vi "ZyklussteuerungGV-01-17.vi"(0 "Traps/MachKoeff0":dbl[](array[numeric]), 1 "DIOsNummern":cluster{"DIOsMod2BNr":i32[]}[](array[cluster]), 2 "error in":errorcluster, 5 "Traps/MachKoeff1":dbl[](array[numeric]), 7 "ServosWarmHigh (us)KaltHigh(us)":T1, 9 "Traps/MachKoeff2":dbl[](array[numeric]), 11 "Schieberegister":T2, 12 "Zeitpunkte/Setpoints":T4 {"FPGAPID"."proportional gain (Kc)" format="%.11g"; "FPGAPID"."integral gain (Kc*Ts/Ti)" format="%.11g"; "FPGAPID"."derivative gain (Kc*Td/Ts)" format="%.11g"}, 13 "FPGA VI Reference In":refnum<k20>, 14 "MachKoeffs":T3) -> (4 "Schieberegister":T2, 8 "error out":errorcluster)   [LabVIEW 2010]
uses:
  <vilib>/rvi/interface/nirviReadWriteControl/nirviReadWriteControl.xnode
  C:/Users/HAGAR-IV/Desktop/Zeugs/markus/version feb 2012/FPGA Bitfiles/pertrasgcfpga2_FPGATarget_FPGA-Programm-01_A75D3647.lvbitx
  C:/Users/HAGAR-IV/Desktop/Zeugs/Johnny/pertrasgc fpga/FPGA-Programm-01-17.vi
  <vilib>/rvi/interface/common/niFpgaNodeNameForErrorReporting.ctl
  <vilib>/rvi/errors/niLvFpgaWhatHappensToTopLevelVI.ctl
  GVZwangs.vi
  GVHeizenLH.vi
  GVZeitenZyklen.vi
  GVZwangsMPV.vi
  GVZwangsMPVPos.vi
  GVVentilposition.vi
  GVHorstSP.vi
  <vilib>/Utility/error.llb/Error Cluster From Error Code.vi
  <vilib>/rvi/errors/niLvFpgaAdjustHostInterfaceError.vi
  NiFpgaLv.dll
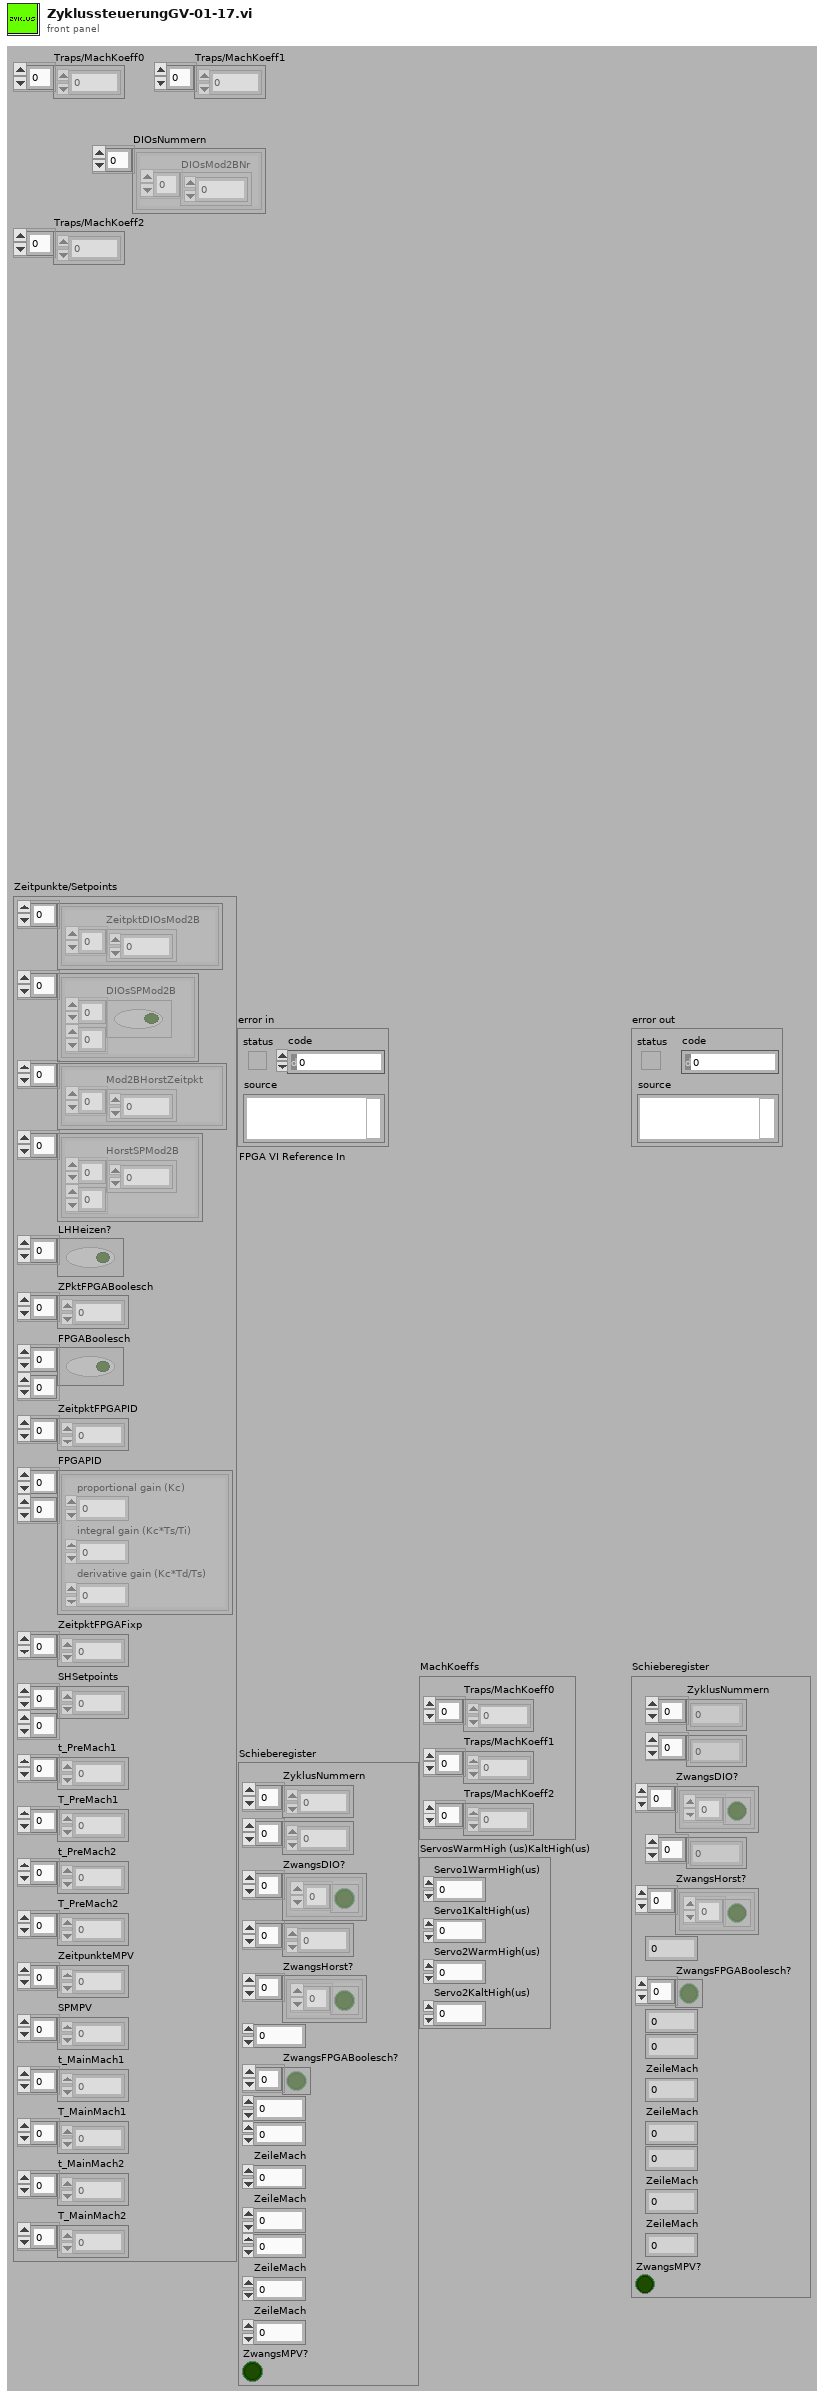
[diagram p1: front panel]
types:
  T1 = cluster{"Servo1WarmHigh(us)":u32, "Servo1KaltHigh(us)":u32, "Servo2WarmHigh(us)":u32, "Servo2KaltHigh(us)":u32}
  T2 = cluster{"ZyklusNummern":i32[], i32[], "ZwangsDIO?":cluster{bool[]}[], i32[], "ZwangsHorst?":cluster{bool[]}[], i32, "ZwangsFPGABoolesch?":bool[], i32, i32, "ZeileMach":i32, "ZeileMach":i32, i32, "ZeileMach":i32, "ZeileMach":i32, "ZwangsMPV?":bool}
  T3 = cluster{"Traps/MachKoeff0":dbl[], "Traps/MachKoeff1":dbl[], "Traps/MachKoeff2":dbl[]}
  T4 = cluster{cluster{"ZeitpktDIOsMod2B":dbl[]}[], cluster{"DIOsSPMod2B":bool[][]}[], cluster{"Mod2BHorstZeitpkt":dbl[]}[], cluster{"HorstSPMod2B":dbl[][]}[], "LHHeizen?":bool[], "ZPktFPGABoolesch":dbl[], "FPGABoolesch":bool[][], "ZeitpktFPGAPID":dbl[], "FPGAPID":cluster{"proportional gain (Kc)":fxp<+/-,16,8>, "integral gain (Kc*Ts/Ti)":fxp<+/-,16,8>, "derivative gain (Kc*Td/Ts)":fxp<+/-,16,8>}[][], "ZeitpktFPGAFixp":dbl[], "SHSetpoints":dbl[][], "t_PreMach1":dbl[], "T_PreMach1":dbl[], "t_PreMach2":dbl[], "T_PreMach2":dbl[], "ZeitpunkteMPV":dbl[], "SPMPV":i32[], "t_MainMach1":dbl[], "T_MainMach1":dbl[], "t_MainMach2":dbl[], "T_MainMach2":dbl[]}
  T5 = cluster{"proportional gain (Kc)":fxp<+/-,16,8>, "integral gain (Kc*Ts/Ti)":fxp<+/-,16,8>, "derivative gain (Kc*Td/Ts)":fxp<+/-,16,8>}[][]
  T6 = typedef "niFpgaNodeNameForErrorReporting.ctl" = enum16{"Open FPGA VI Reference", "Read/Write Control", "Invoke Method: Abort", "Invoke Method: Acknowledge IRQ", "Invoke Method: Download", "Invoke Method: FIFO.Configure", "Invoke Method: FIFO.Read", "Invoke Method: FIFO.Start", "Invoke Method: FIFO.Stop", "Invoke Method: FIFO.Write", "Invoke Method: Reset", "Invoke Method: Run", "Invoke Method: Wait on IRQ", "Close FPGA VI Reference"}
  T7 = typedef "niLvFpgaWhatHappensToTopLevelVI.ctl" = enum16{"top level VI scripted behind XNode", "top level VI inlined behind XNode"}
  T8 = cluster{"[0]":bool, "[1]":bool, "[2]":bool, "[3]":bool, "[4]":bool, "[5]":bool, "[6]":bool, "[7]":bool, "[8]":bool, "[9]":bool, "[10]":bool, "[11]":bool, "[12]":bool, "[13]":bool, "[14]":bool, "[15]":bool, "[16]":bool, "[17]":bool, "[18]":bool, "[19]":bool, "[20]":bool, "[21]":bool, "[22]":bool, "[23]":bool, "[24]":bool, "[25]":bool, "[26]":bool, "[27]":bool, "[28]":bool, "[29]":bool, "[30]":bool, "[31]":bool}
  T9 = cluster{"[0]":bool, "[1]":bool, "[2]":bool, "[3]":bool, "[4]":bool, "[5]":bool, "[6]":bool, "[7]":bool, "[8]":bool, "[9]":bool}
  T10 = cluster{"proportional gain (Kc)":fxp<+/-,16,8>, "integral gain (Kc*Ts/Ti)":fxp<+/-,16,8>, "derivative gain (Kc*Td/Ts)":fxp<+/-,16,8>}[]
  T11 = cluster{"FPGAPID[0]":cluster{"proportional gain (Kc)":fxp<+/-,16,8>, "integral gain (Kc*Ts/Ti)":fxp<+/-,16,8>, "derivative gain (Kc*Td/Ts)":fxp<+/-,16,8>}, "FPGAPID[1]":cluster{"proportional gain (Kc)":fxp<+/-,16,8>, "integral gain (Kc*Ts/Ti)":fxp<+/-,16,8>, "derivative gain (Kc*Td/Ts)":fxp<+/-,16,8>}, "FPGAPID[2]":cluster{"proportional gain (Kc)":fxp<+/-,16,8>, "integral gain (Kc*Ts/Ti)":fxp<+/-,16,8>, "derivative gain (Kc*Td/Ts)":fxp<+/-,16,8>}, "FPGAPID[3]":cluster{"proportional gain (Kc)":fxp<+/-,16,8>, "integral gain (Kc*Ts/Ti)":fxp<+/-,16,8>, "derivative gain (Kc*Td/Ts)":fxp<+/-,16,8>}, "FPGAPID[4]":cluster{"proportional gain (Kc)":fxp<+/-,16,8>, "integral gain (Kc*Ts/Ti)":fxp<+/-,16,8>, "derivative gain (Kc*Td/Ts)":fxp<+/-,16,8>}, "FPGAPID[5]":cluster{"proportional gain (Kc)":fxp<+/-,16,8>, "integral gain (Kc*Ts/Ti)":fxp<+/-,16,8>, "derivative gain (Kc*Td/Ts)":fxp<+/-,16,8>}}
  T12 = cluster{"proportional gain (Kc)":fxp<+/-,16,8>, "integral gain (Kc*Ts/Ti)":fxp<+/-,16,8>, "derivative gain (Kc*Td/Ts)":fxp<+/-,16,8>}
  T13 = cluster{"USetp [V]Mach1":fxp<+/-,16,6>, "[1]":fxp<+/-,16,4>, "[2]":fxp<+/-,16,4>, "[3]":fxp<+/-,16,4>, "[4]":fxp<+/-,16,4>, "[5]":fxp<+/-,16,4>, "[6]":fxp<+/-,16,4>, "[7]":fxp<+/-,16,4>, "[8]":fxp<+/-,16,4>}
  T14 = cluster{"SpannungenSH[V][0]":fxp<+/-,16,4>, "SpannungenSH[V][1]":fxp<+/-,16,4>, "SpannungenSH[V][2]":fxp<+/-,16,4>, "SpannungenSH[V][3]":fxp<+/-,16,4>}
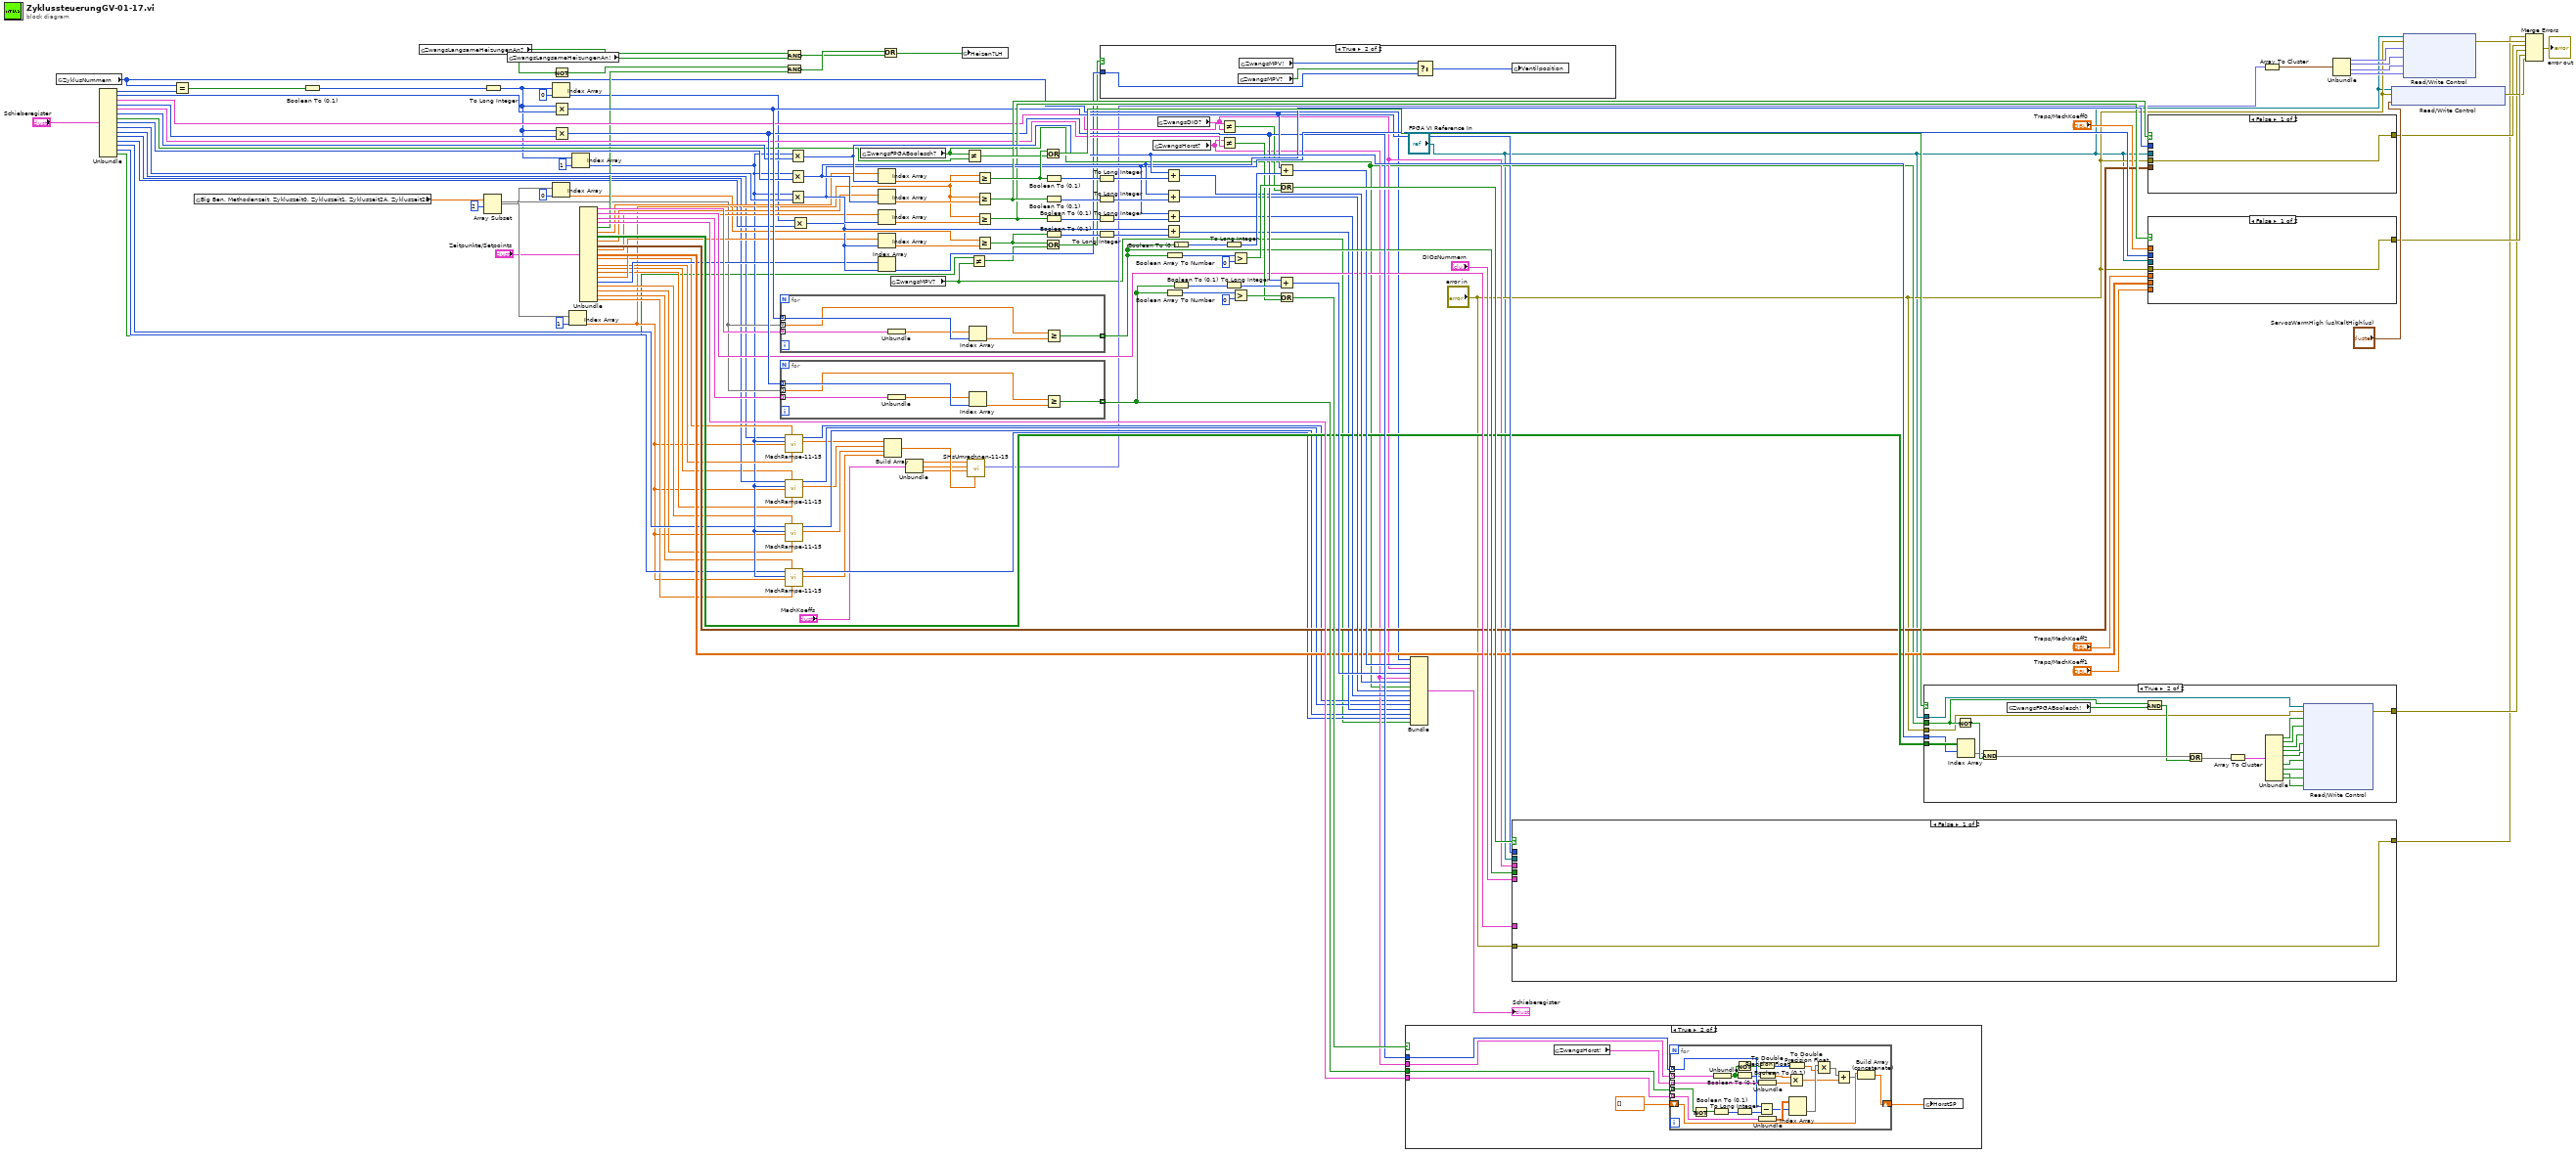
[diagram p0: block diagram]
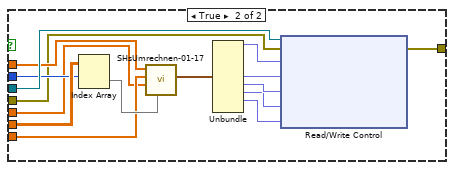
[diagram p4: hidden frame]
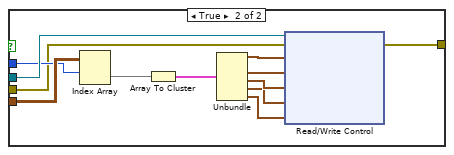
[diagram p5: hidden frame]
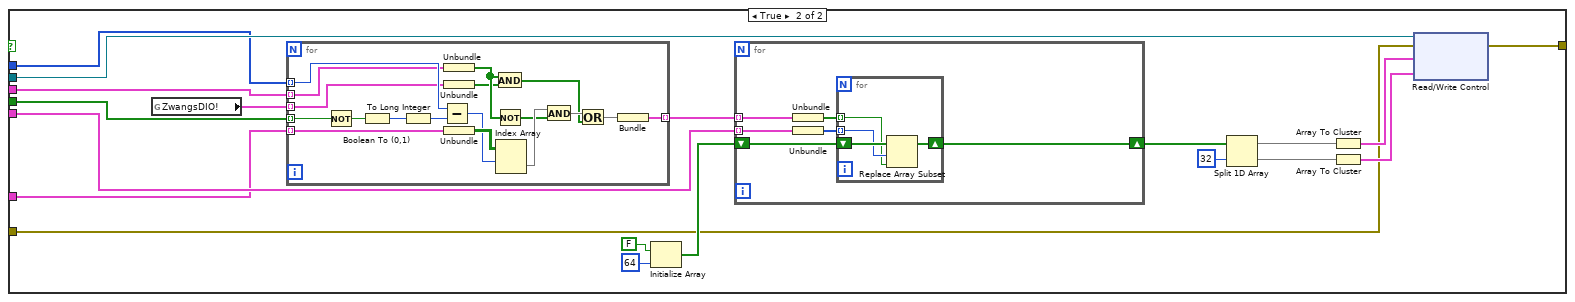
[diagram p7: hidden frame]
diagram:
  n1 = global read "GVZeitenZyklen.vi" "ZyklusNummern"() -> (w59:i32[])
  n2 = Unbundle("Schieberegister") -> ("ZyklusNummern"=w103:i32[], w102:i32[], "ZwangsDIO?"=w101:cluster{bool[]}[], w100:i32[], "ZwangsHorst?"=w99:cluster{bool[]}[], w98:i32, "ZwangsFPGABoolesch?"=w97:bool[], w96:i32, w95:i32, "ZeileMach"=w36:i32, "ZeileMach"=w51:i32, w62:i32, "ZeileMach"=w49:i32, "ZeileMach"=w48:i32, "ZwangsMPV?"=w14:bool)
  n3 = Equal?(x=w59, y=w103) -> (x = y?=w146:bool[])
  n4 = global read "GVZeitenZyklen.vi" "Big Ben, Methodenzeit, Zykluszeit0, Zykluszeit1, Zykluszeit2A, Zykluszeit2B"() -> (w57:dbl[])
  n5 = Boolean To (0,1)(Boolean=w146) -> (0, 1=w145:i16[])
  n6 = global read "GVZwangs.vi" "ZwangsLangsameHeizungenAn?"() -> (w76:bool[])
  n7 = Array Subset(array=w57, index=2 ("Index")) -> (w56:dbl[])  [unwired: 1 in]
  n8 = To Long Integer(number=w145) -> (32bit integer=w72:i32[])
  n9 = global read "GVZwangs.vi" "ZwangsLangsameHeizungenAn!"() -> (w75:bool[])
  n10 = Index Array(array=w72, index=0 ("Index")) -> (element=w70:i32)
  n11 = Index Array(array=w56, index=0 ("Index")) -> (element=w67:dbl)
  n12 = Not(x=w76) -> (.not. x?=w114:bool[])
  n13 = Multiply(x=w72, y=w102) -> (x*y=w111:i32[])
  n14 = Multiply(x=w72, y=w100) -> (x*y=w108:i32[])
  n15 = Index Array(array=w56, index=1 ("Index")) -> (element=w37:dbl)
  n16 = Index Array(array=w72, index=1 ("Index")) -> (element=w50:i32)
  n17 = Unbundle("Zeitpunkte/Setpoints") -> (w89:cluster{"ZeitpktDIOsMod2B":dbl[]}[], w88:cluster{"DIOsSPMod2B":bool[][]}[], w87:cluster{"Mod2BHorstZeitpkt":dbl[]}[], w86:cluster{"HorstSPMod2B":dbl[][]}[], "LHHeizen?"=w85:bool[], "ZPktFPGABoolesch"=w84:dbl[], "FPGABoolesch"=w83:bool[][], "ZeitpktFPGAPID"=w82:dbl[], "FPGAPID"=w81:T5, "ZeitpktFPGAFixp"=w80:dbl[], "SHSetpoints"=w79:dbl[][], "t_PreMach1"=w54:dbl[], "T_PreMach1"=w53:dbl[], "t_PreMach2"=w47:dbl[], "T_PreMach2"=w46:dbl[], "ZeitpunkteMPV"=w61:dbl[], "SPMPV"=w60:i32[], "t_MainMach1"=w45:dbl[], "T_MainMach1"=w44:dbl[], "t_MainMach2"=w43:dbl[], "T_MainMach2"=w42:dbl[])
  n18 = for {
    tunnel: w111 -> [w152] mode=indexing
    tunnel: w56 -> [w151] mode=indexing
    tunnel: [w150] -> w105 mode=indexing
    tunnel: w89 -> [w148] mode=indexing
    n19 = Unbundle(w148) -> ("ZeitpktDIOsMod2B"=w147:dbl[])
    n20 = Index Array(array=w147, index=w152) -> (element=w149:dbl)
    n21 = Greater Or Equal?(x=w151, y=w149) -> (x >= y?=w150:bool)
  }
  n22 = for {
    tunnel: w108 -> [w158] mode=indexing
    tunnel: w56 -> [w157] mode=indexing
    tunnel: w87 -> [w154] mode=indexing
    tunnel: [w155] -> w109 mode=indexing
    n23 = Unbundle(w154) -> ("Mod2BHorstZeitpkt"=w153:dbl[])
    n24 = Index Array(array=w153, index=w158) -> (element=w156:dbl)
    n25 = Greater Or Equal?(x=w157, y=w156) -> (x >= y?=w155:bool)
  }
  n26 = call "MachRampe-11-15.vi"("T_Mach"=w53, "t_Mach"=w54, "ZykluszeitMod1"=w37, "gleicherZyklus?"=w50, "ZeileMach"=w36) -> ("T_Mach"=w35:dbl, "ZeileMach"=w52:i32)  [unwired: 5 in]
  n27 = call "MachRampe-11-15.vi"("T_Mach"=w46, "t_Mach"=w47, "ZykluszeitMod1"=w37, "gleicherZyklus?"=w50, "ZeileMach"=w51) -> ("T_Mach"=w34:dbl, "ZeileMach"=w41:i32)  [unwired: 5 in]
  n28 = call "MachRampe-11-15.vi"("T_Mach"=w44, "t_Mach"=w45, "ZykluszeitMod1"=w37, "gleicherZyklus?"=w50, "ZeileMach"=w49) -> ("T_Mach"=w33:dbl, "ZeileMach"=w40:i32)  [unwired: 5 in]
  n29 = call "MachRampe-11-15.vi"("T_Mach"=w42, "t_Mach"=w43, "ZykluszeitMod1"=w37, "gleicherZyklus?"=w50, "ZeileMach"=w48) -> ("T_Mach"=w32:dbl, "ZeileMach"=w39:i32)  [unwired: 5 in]
  n30 = And(x=w76, y=w75) -> (x .and. y?=w112:bool[])
  n31 = And(x=w114, y=w85) -> (x .and. y?=w113:bool[])
  n32 = Multiply(x=w50, y=w98) -> (x*y=w125:i32)
  n33 = Multiply(x=w50, y=w96) -> (x*y=w120:i32)
  n34 = Multiply(x=w50, y=w95) -> (x*y=w116:i32)
  n35 = Multiply(x=w70, y=w62) -> (x*y=w64:i32)
  n36 = global read "GVZwangs.vi" "ZwangsFPGABoolesch?"() -> (w73:bool[])
  n37 = Index Array(array=w84, index=w125) -> (element=w131:dbl)
  n38 = Index Array(array=w82, index=w120) -> (element=w124:dbl)
  n39 = Index Array(array=w80, index=w116) -> (element=w119:dbl)
  n40 = Index Array(array=w61, index=w64) -> (element=w68:dbl)
  n41 = Index Array(array=w60, index=w64) -> (element=w17:i32)
  n42 = Or(x=w113, y=w112) -> (x .or. y?=w74:bool[])
  n43 = Build Array(w35, w34, w33, w32) -> (w31:dbl[])
  n44 = global read "GVZwangsMPV.vi" "ZwangsMPV?"() -> (w15:bool)
  n45 = Unbundle("MachKoeffs") -> ("Traps/MachKoeff0"=w26:dbl[], "Traps/MachKoeff1"=w25:dbl[], "Traps/MachKoeff2"=w24:dbl[])
  n46 = global write "GVHeizenLH.vi" "Heizen?LH"(w74) -> ()
  n47 = Not Equal?(x=w73, y=w97) -> (x != y?=w127:bool)
  n48 = call "SHsUmrechnen-11-15.vi"("TemperaturenSH[V]"=w31, "Traps/MachKoeff2"=w24, "Traps/MachKoeff1"=w25, "Traps/MachKoeff0"=w26) -> ("SpannungenSH[V]"=w23:fxp<+/-,16,4>[])  [unwired: 6 in, 1 out]
  n49 = Not Equal?(x=w14, y=w15) -> (x != y?=w13:bool)
  n50 = Greater Or Equal?(x=w37, y=w131) -> (x >= y?=w128:bool)
  n51 = Greater Or Equal?(x=w37, y=w124) -> (x >= y?=w121:bool)
  n52 = Greater Or Equal?(x=w37, y=w119) -> (x >= y?=w115:bool)
  n53 = Greater Or Equal?(x=w67, y=w68) -> (x >= y?=w12:bool)
  n54 = Or(x=w128, y=w127) -> (x .or. y?=w126:bool)
  n55 = Or(x=w12, y=w13) -> (x .or. y?=w11:bool)
  n56 = Boolean To (0,1)(Boolean=w128) -> (0, 1=w130:i16)
  n57 = Boolean To (0,1)(Boolean=w121) -> (0, 1=w123:i16)
  n58 = Boolean To (0,1)(Boolean=w115) -> (0, 1=w118:i16)
  n59 = Boolean To (0,1)(Boolean=w12) -> (0, 1=w66:i16)
  n60 = To Long Integer(number=w130) -> (32bit integer=w129:i32)
  n61 = To Long Integer(number=w123) -> (32bit integer=w122:i32)
  n62 = To Long Integer(number=w118) -> (32bit integer=w117:i32)
  n63 = To Long Integer(number=w66) -> (32bit integer=w65:i32)
  n64 = case shown="True" w11 {
    tunnel: w17 -> [_ w160]
    frame False {
    }
    frame True {
      n65 = global read "GVZwangsMPV.vi" "ZwangsMPV?"() -> (w162:bool)
      n66 = global read "GVZwangsMPVPos.vi" "ZwangsMPV!"() -> (w161:i32)
      n67 = Select(t=w161, s=w162, f=w160) -> (s? t:f=w159:i32)
      n68 = global write "GVVentilposition.vi" "Ventilposition"(w159) -> ()
    }
  }
  n69 = global read "GVZwangs.vi" "ZwangsHorst?"() -> (w77:cluster{bool[]}[])
  n70 = global read "GVZwangs.vi" "ZwangsDIO?"() -> (w78:cluster{bool[]}[])
  n71 = Add(x=w125, y=w129) -> (x+y=w92:i32)
  n72 = Add(x=w120, y=w122) -> (x+y=w91:i32)
  n73 = Add(x=w116, y=w117) -> (x+y=w90:i32)
  n74 = Add(x=w64, y=w65) -> (x+y=w63:i32)
  n75 = Boolean Array To Number(Boolean array=w105) -> (number=w142:u32)
  n76 = Boolean Array To Number(Boolean array=w109) -> (number=w136:u32)
  n77 = Boolean To (0,1)(Boolean=w105) -> (0, 1=w144:i16[])
  n78 = Boolean To (0,1)(Boolean=w109) -> (0, 1=w138:i16[])
  n79 = Not Equal?(x=w101, y=w78) -> (x != y?=w106:bool)
  n80 = Not Equal?(x=w77, y=w99) -> (x != y?=w107:bool)
  n81 = To Long Integer(number=w144) -> (32bit integer=w143:i32[])
  n82 = To Long Integer(number=w138) -> (32bit integer=w137:i32[])
  n83 = Greater?(x=w142, y=u32 0) -> (0:w139:bool)
  n84 = Greater?(x=w136, y=u32 0) -> (0:w134:bool)
  n85 = Add(x=w111, y=w143) -> (x+y=w94:i32[])
  n86 = Or(x=w139, y=w106) -> (x .or. y?=w140:bool)
  n87 = Add(x=w108, y=w137) -> (x+y=w93:i32[])
  n88 = Or(x=w134, y=w107) -> (x .or. y?=w110:bool)
  n89 = case shown="True" w110 {
    tunnel: w86 -> [_ w166]
    tunnel: w77 -> [_ w167]
    tunnel: w109 -> [_ w169]
    tunnel: w108 -> [_ w168]
    frame False {
    }
    frame True {
      n90 = global read "GVZwangs.vi" "ZwangsHorst!"() -> (w164:cluster{dbl[]}[])
      n91 = for {
        tunnel: w169 -> [w189] mode=indexing
        tunnel: w168 -> [w186] mode=indexing
        tunnel: w167 -> [w192] mode=indexing
        tunnel: w166 -> [w190] mode=indexing
        tunnel: w164 -> [w191] mode=indexing
        shift-right: [w170] -> w163
        shift-left: dbl[] [] -> [w172]
        n92 = Not(x=w189) -> (.not. x?=w188:bool)
        n93 = Boolean To (0,1)(Boolean=w188) -> (0, 1=w187:i16)
        n94 = Unbundle(w192) -> (w179:bool[])
        n95 = Not(x=w179) -> (.not. x?=w182:bool[])
        n96 = Boolean To (0,1)(Boolean=w179) -> (0, 1=w180:i16[])
        n97 = To Long Integer(number=w187) -> (32bit integer=w185:i32)
        n98 = Subtract(x=w186, y=w185) -> (x-y=w183:i32)
        n99 = Boolean To (0,1)(Boolean=w182) -> (0, 1=w181:i16[])
        n100 = To Double Precision Float(number=w180) -> (double precision float=w176:dbl[])
        n101 = Unbundle(w191) -> (w175:dbl[])
        n102 = Unbundle(w190) -> ("HorstSPMod2B"=w184:dbl[][])
        n103 = Multiply(x=w176, y=w175) -> (x*y=w173:dbl[])
        n104 = To Double Precision Float(number=w181) -> (double precision float=w177:dbl[])
        n105 = Index Array(array=w184, index (row)=w183) -> (element=w178:dbl[])  [unwired: 1 in]
        n106 = Multiply(x=w178, y=w177) -> (x*y=w174:dbl[])
        n107 = Add(x=w174, y=w173) -> (x+y=w171:dbl[])
        n108 = Build Array (concatenate)(w172, w171) -> (w170:dbl[])
      }
      n109 = global write "GVHorstSP.vi" "HorstSP"(w163) -> ()
    }
  }
  n110 = Bundle("ZyklusNummern"=w59, w94, "ZwangsDIO?"=w78, w93, "ZwangsHorst?"=w77, w92, "ZwangsFPGABoolesch?"=w73, w91, w90, "ZeileMach"=w52, "ZeileMach"=w41, w63, "ZeileMach"=w40, "ZeileMach"=w39, "ZwangsMPV?"=w15) -> (→"Schieberegister":T2)  [unwired: 1 in]
  n111 = case shown="False" w140 {
    tunnel: w111 -> [_ w208]
    tunnel: w78 -> [_ w205]
    tunnel: "DIOsNummern" -> [_ w212]
    tunnel: "FPGA VI Reference In" -> [_ w211]
    tunnel: w88 -> [_ w206]
    tunnel: w105 -> [_ w207]
    tunnel: "error in" -> [w193 w195]
    tunnel: [w193 w194] -> w3
    frame False {
    }
    frame True {
      n112 = global read "GVZwangs.vi" "ZwangsDIO!"() -> (w196:cluster{bool[]}[])
      n113 = for {
        tunnel: w208 -> [w227] mode=indexing
        tunnel: w207 -> [w226] mode=indexing
        tunnel: w206 -> [w225] mode=indexing
        tunnel: w205 -> [w224] mode=indexing
        tunnel: w196 -> [w223] mode=indexing
        tunnel: [w213] -> w204 mode=indexing
        n114 = Not(x=w226) -> (.not. x?=w229:bool)
        n115 = Boolean To (0,1)(Boolean=w229) -> (0, 1=w228:i16)
        n116 = To Long Integer(number=w228) -> (32bit integer=w230:i32)
        n117 = Subtract(x=w227, y=w230) -> (x-y=w221:i32)
        n118 = Unbundle(w224) -> (w218:bool[])
        n119 = Unbundle(w223) -> (w217:bool[])
        n120 = Unbundle(w225) -> ("DIOsSPMod2B"=w222:bool[][])
        n121 = And(x=w218, y=w217) -> (x .and. y?=w215:bool[])
        n122 = Not(x=w218) -> (.not. x?=w219:bool[])
        n123 = Index Array(array=w222, index (row)=w221) -> (element=w220:bool[])  [unwired: 1 in]
        n124 = And(x=w220, y=w219) -> (x .and. y?=w216:bool[])
        n125 = Or(x=w216, y=w215) -> (x .or. y?=w214:bool[])
        n126 = Bundle(w214) -> (w213:cluster{bool[]})  [unwired: 1 in]
      }
      n127 = Initialize Array(FALSE, 64 ("Dimension")) -> (w197:bool[])
      n128 = for {
        tunnel: w204 -> [w305] mode=indexing
        tunnel: w212 -> [w307] mode=indexing
        shift-right: [w308] -> w209
        shift-left: w197 -> [w309]
        n129 = Unbundle(w305) -> (w304:bool[])
        n130 = Unbundle(w307) -> ("DIOsMod2BNr"=w306:i32[])
        n131 = for {
          tunnel: w304 -> [w311] mode=indexing
          tunnel: w306 -> [w312] mode=indexing
          shift-right: [w310] -> w308
          shift-left: w309 -> [w313]
          n132 = Replace Array Subset(array=w313, new element=w311, index=w312) -> (w310:bool[])
        }
      }
      n133 = Split 1D Array(array=w209, index=32 ("Länge")) -> (first subarray=w203:bool[], second subarray=w201:bool[])
      n134 = Array To Cluster(array=w203) -> (cluster=w202:T8)
      n135 = Array To Cluster(array=w201) -> (cluster=w200:T8)
      n136 = xnode "Read/Write Control"("FPGA VI Reference In"=w211, "error in"=w195, "Mod5/DIO"=w202, "Mod6/DIO"=w200) -> ("error out"=w194:errorcluster)  [unwired: 1 out]
    }
  }
  n137 = case shown="True" w126 {
    tunnel: w125 -> [_ w327]
    tunnel: w73 -> [_ w332]
    tunnel: w83 -> [_ w336]
    tunnel: "FPGA VI Reference In" -> [_ w329]
    tunnel: "error in" -> [w314 w316]
    tunnel: [w314 w315] -> w7
    frame False {
    }
    frame True {
      n138 = Not(x=w332) -> (.not. x?=w335:bool[])
      n139 = Index Array(array=w336, index (row)=w327) -> (element=w334:bool[])  [unwired: 1 in]
      n140 = And(x=w334, y=w335) -> (x .and. y?=w333:bool[])
      n141 = global read "GVZwangs.vi" "ZwangsFPGABoolesch!"() -> (w326:bool[])
      n142 = And(x=w332, y=w326) -> (x .and. y?=w331:bool[])
      n143 = Or(x=w333, y=w331) -> (x .or. y?=w330:bool[])
      n144 = Array To Cluster(array=w330) -> (cluster=w328:T9)
      n145 = Unbundle(w328) -> ("[0]"=w325:bool, "[1]"=w324:bool, "[2]"=w323:bool, "[3]"=w322:bool, "[4]"=w321:bool, "[6]"=w320:bool, "[7]"=w319:bool, "[8]"=w318:bool, "[9]"=w317:bool)  [unwired: 1 out]
      n146 = xnode "Read/Write Control"("FPGA VI Reference In"=w329, "error in"=w316, "Servo1An?"=w325, "Servo2An?"=w324, "ServoTrap1kalt"=w323, "ServoTrap2kalt"=w322, "Heizen?Trap1"=w321, "Heizen?PreMach1"=w320, "Heizen?PreMach2"=w319, "Heizen?MainMach1"=w318, "Heizen?MainMach2"=w317) -> ("error out"=w315:errorcluster)  [unwired: 1 out]
    }
  }
  n147 = case shown="False" w121 {
    tunnel: "FPGA VI Reference In" -> [_ w555]
    tunnel: w81 -> [_ w554]
    tunnel: w120 -> [_ w548]
    tunnel: "error in" -> [w543 w545]
    tunnel: [w543 w544] -> w6
    frame False {
    }
    frame True {
      n148 = Index Array(array=w554, index (row)=w548) -> (element=w553:T10)  [unwired: 1 in]
      n149 = Array To Cluster(array=w553) -> (cluster=w552:T11)
      n150 = Unbundle(w552) -> ("FPGAPID[0]"=w551:T12, "FPGAPID[2]"=w550:T12, "FPGAPID[3]"=w549:T12, "FPGAPID[4]"=w547:T12, "FPGAPID[5]"=w546:T12)  [unwired: 1 out]
      n151 = xnode "Read/Write Control"("FPGA VI Reference In"=w555, "error in"=w545, "PIDTrap1"=w551, "PIDPreMach1"=w550, "PIDPreMach2"=w549, "PIDMainMach1"=w547, "PIDMainMach2"=w546) -> ("error out"=w544:errorcluster)  [unwired: 1 out]
    }
  }
  n152 = case shown="False" w115 {
    tunnel: w116 -> [_ w716]
    tunnel: w79 -> [_ w718]
    tunnel: "FPGA VI Reference In" -> [_ w717]
    tunnel: "Traps/MachKoeff2" -> [_ w706]
    tunnel: "Traps/MachKoeff1" -> [_ w707]
    tunnel: "Traps/MachKoeff0" -> [_ w708]
    tunnel: "error in" -> [w703 w705]
    tunnel: [w703 w704] -> w9
    frame False {
    }
    frame True {
      n153 = Index Array(array=w718, index (row)=w716) -> (element=w709:dbl[])  [unwired: 1 in]
      n154 = call "SHsUmrechnen-01-17.vi"("TemperaturenSH[V]"=w709, "Traps/MachKoeff2"=w706, "Traps/MachKoeff1"=w707, "Traps/MachKoeff0"=w708) -> ("Spannungen SH"=w710:T13)  [unwired: 6 in, 1 out]
      n155 = Unbundle(w710) -> ("USetp [V]Mach1"=w715:fxp<+/-,16,6>, "[4]"=w714:fxp<+/-,16,4>, "[5]"=w713:fxp<+/-,16,4>, "[6]"=w712:fxp<+/-,16,4>, "[7]"=w711:fxp<+/-,16,4>)  [unwired: 4 out]
      n156 = xnode "Read/Write Control"("FPGA VI Reference In"=w717, "error in"=w705, "SetpointTrap1"=w715, "Umax[V]PreMach1"=w714, "Umax[V]PreMach2"=w713, "Umax[V]MainMach1"=w712, "Umax[V]MainMach2"=w711) -> ("error out"=w704:errorcluster)  [unwired: 1 out]
    }
  }
  n157 = Array To Cluster(array=w23) -> (cluster=w22:T14)
  n158 = Unbundle(w22) -> ("SpannungenSH[V][0]"=w21:fxp<+/-,16,4>, "SpannungenSH[V][1]"=w20:fxp<+/-,16,4>, "SpannungenSH[V][2]"=w19:fxp<+/-,16,4>, "SpannungenSH[V][3]"=w18:fxp<+/-,16,4>)
  n159 = xnode "Read/Write Control"("FPGA VI Reference In"="FPGA VI Reference In", "error in"="error in", "ServosWarmHigh (us)KaltHigh(us)"="ServosWarmHigh (us)KaltHigh(us)") -> ("error out"=w8:errorcluster)  [unwired: 1 out]
  n160 = xnode "Read/Write Control"("FPGA VI Reference In"="FPGA VI Reference In", "error in"="error in", "USetp[V]PreMach1"=w21, "USetp[V]PreMach2"=w20, "USetp[V]MainMach1"=w19, "USetp[V]MainMach2"=w18) -> ("error out"=w5:errorcluster)  [unwired: 1 out]
  n161 = Merge Errors(w3, w5, w6, w7, w9, w8) -> (→"error out":errorcluster)
